vi "RVC Drive to Pose Maneuver.vi"() -> ()   [LabVIEW 2017]
uses:
  <vilib>/Simulation/Scripting/Companion Diagram/SimConfigNode/SimParams.ctl
  <vilib>/Simulation/Scripting/Companion Diagram/SimConfigNode/_simSolvers.ctl
  <vilib>/Simulation/Implementation/Shared/SIMSCR Execution Mode.ctl
  <vilib>/Simulation/Param Hierarchy/Typedefs/SIMPH Param Control Actions.ctl
  <vilib>/Simulation/Scripting/Editor Utilities/SIM subVI tag data.ctl
  <vilib>/Simulation/Scripting/Editor Utilities/SIM subVI execution type.ctl
  <vilib>/Simulation/Implementation/Shared/NILVSim_ParamChanged.vi
  <vilib>/Simulation/Implementation/Shared/NILVSIM_BeginStep.vi
  <vilib>/Simulation/Utility/Implementation/SIM Time.vi
  <vilib>/Simulation/Utility/Implementation/NILVSim Collector.llb/SIM Collector (vector).vi
  <vilib>/Simulation/SignalArithmetic/Implementation/NILVSim Gain.llb/SIM Gain (scalar).vi
  <vilib>/Simulation/Utility/Implementation/SIM Halt.vi
  <vilib>/Simulation/Utility/Implementation/NILVSim Collector.llb/SIM Collector (scalar).vi
  <vilib>/Simulation/Implementation/Shared/SIM Fire Discrete SubVI.vi
  <vilib>/Simulation/Implementation/Shared/NILVSim_Manager.vi
  <vilib>/Utility/error.llb/Clear Errors.vi
  <vilib>/Simulation/Implementation/Shared/NILVSim_FinalizeModel.vi
  <vilib>/Simulation/Utility/Implementation/NILVSim Collector.llb/NILVSim Collector core (vector).vi
  <vilib>/Simulation/Utility/Implementation/NILVSim Collector.llb/NILVSim Collector core (scalar).vi
  <vilib>/Simulation/Implementation/Shared/SIM Fire Discrete SubVI (Core).vi
  <vilib>/Simulation/Implementation/Shared/SIM Unbundle Sim Info.vi
  <vilib>/Simulation/Implementation/Shared/NILVSim_Initialize.vi
  <vilib>/Simulation/Utility/Implementation/NILVSim Get Time and IsAcceptedStep.vi
  subVIs/2D Animation.vi
  subVIs/RVC To Polar.vi
  subVIs/2D Animate Rotating Wheel.vi
  <vilib>/Simulation/Implementation/Shared/SIMSH Read Queue.vi
  <vilib>/Simulation/Implementation/Shared/NILVSim_GetModelError.vi
  <vilib>/Simulation/Implementation/Shared/SIM Bundle Sim Info.vi
  <vilib>/Simulation/Scripting/Companion Diagram/SimConfigNode/SimDog.xnode
  SIM Bicycle.vi
  <vilib>/Simulation/Implementation/XNodeFramework/SimXNode/SimX.xnode
  <vilib>/Simulation/Implementation/Shared/NI_SIM_Implementation.lvlib
panel:
  out "Velocity":cluster{"Time":dbl[], "Signal":dbl[]}[](graph)
  out "Steering":cluster{"Time":dbl[], "Signal":dbl[]}[](graph)
  out "velocity":dbl(knob)=1.0 scale=0.0..10.0
  out "Drive to Pose":cluster{"Time":dbl[], "Signal":dbl[]}[](graph)
  out "Position":cluster{"x":dbl, "y":dbl, "theta":dbl}
  out "Steering Angle":dbl format="%.2f"
  out "Steering Angle":picture
  in  "Pose":dbl[](array[numeric])=[5.0, 5.0, 1.57]
  out "Map Floor":picture
  # "Velocity"
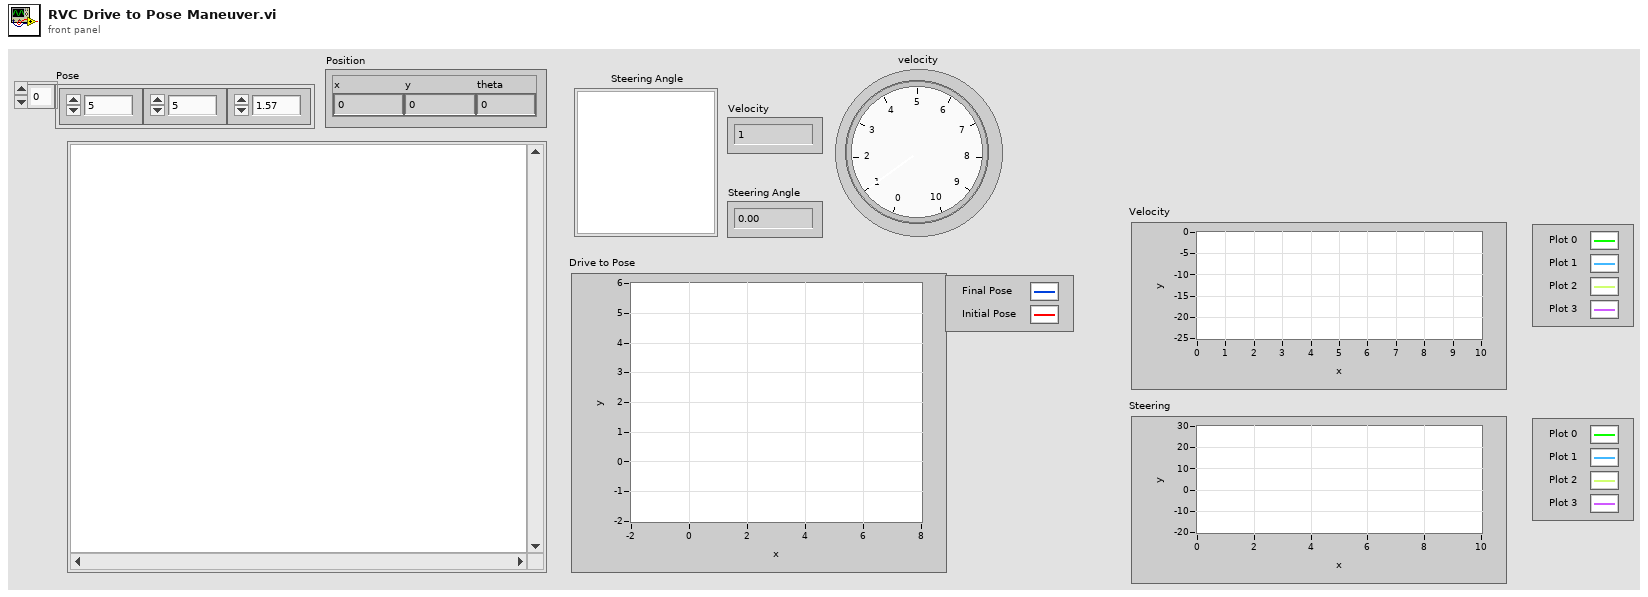
[diagram p1: front panel]
types:
  T1 = typedef "SIMSCR Execution Mode.ctl" = enum16{"Simulate to Completion", "Single Time-Step Simulation (Fixed Step Only)"}
  T2 = typedef "SIMPH Param Control Actions.ctl" = enum16{"get params", "set params"}
  T3 = typedef "SIM subVI tag data.ctl" = cluster{"period":dbl, "skew":dbl, "Simulation execution type":T4}
  T4 = typedef "SIM subVI execution type.ctl" = enum16{"Function call", "Discrete", "Continuous", "Initialization only", "Final step only"}
  T5 = cluster{"SIMSH Sim Time":dbl, "Build Array 2":cluster{"appended array":dbl[]}, "Divide 2":cluster{"x/y":dbl}, "Sine & Cosine":cluster{"sin(x)":dbl, "cos(x)":dbl}, "initial condition":dbl[], "Index Array 4":cluster{"element":dbl}, "vel limit":cluster{"output":dbl}, "steering angle limit":cluster{"output":dbl}, "acceleration limit":cluster{"output":dbl}, "Product":cluster{"Result":dbl[]}, "Build Array":cluster{"appended array":dbl[]}, "Integrator":cluster{"output":dbl[]}}
  T6 = typedef "SimParams.ctl" = cluster{"Initial Time (s)":dbl, "Final Time (s)":dbl, "Step Size (s)":dbl, "ODE Solver":T7, "Minimum Step Size (s)":dbl, "Maximum Step Size (s)":dbl, "Relative Tolerance":dbl, "Absolute Tolerance":dbl, "Software Timing":bool, "Initial Step Size (s)":dbl, "Automatic Fixed Step Size?":bool, "Automatic Discrete Step Size?":bool, "Discrete Step Size (s)":dbl, "Calculate using Time Step":bool, "Solver Wired?":bool, "Prev.Frm.Expected End":u64, "Prev.Frm.Actual End":u64, "Prev.Frm.Finished Late?":bool, "Prev.Iter.Expected End":u64, "Prev.Iter.Actual End":u64, "Prev.Iter.Finished Late?":bool, "Expected Iteration Start":u64, "Actual Iteration Start":u64, "Expected Frame Start":u64, "Actual Frame Start":u64, "Source Name":string, "Name":string, "Period":i64, "Deadline":i64, "Offset":i64, "Start":i64, "Priority":i32, "Timeout":i32, "Processor":i32, "Mode":enum32{"No Change", "Process missed periods, maintain original phase", "Discard missed periods, maintain original phase", "Process missed periods, ignore original phase", "Discard missed periods, ignore original phase"}, "Wakeup reason":enum32{"Normal", "Aborted", "Asynchronous wakeup", "Timing source error", "Timed loop error", "Timeout"}, "Error":errorcluster, "Source Type":string, "Secondary Source Type":string, "Global End Time":u64, "Global Start Time":u64, "Full Solver Reset":bool, "Execution Mode":T1, "Nan/Inf Check":bool, "Custom Solver Library":string, "Solver Is Variable":bool, "custom solver name":string, "Signal Collection Decimation":u32}
  T7 = typedef "_simSolvers.ctl" = enum16{"Runge-Kutta 1 (Euler)", "Runge-Kutta 2", "Runge-Kutta 3", "Runge-Kutta 4", "Runge-Kutta 23 (variable)", "Runge-Kutta 45 (variable)", "BDF (variable)", "Adams-Moulton (variable)", "Rosenbrock (variable)", "Discrete States Only", "SDIRK 4 (variable)", "Radau 5 (variable)", "Radau 9 (variable)", "Radau 13 (variable)", "Radau [Variable Order] (variable)", "Gear's Method (variable)", "Linearizer", "State Query", "Trim Eval", "Custom Solver"}
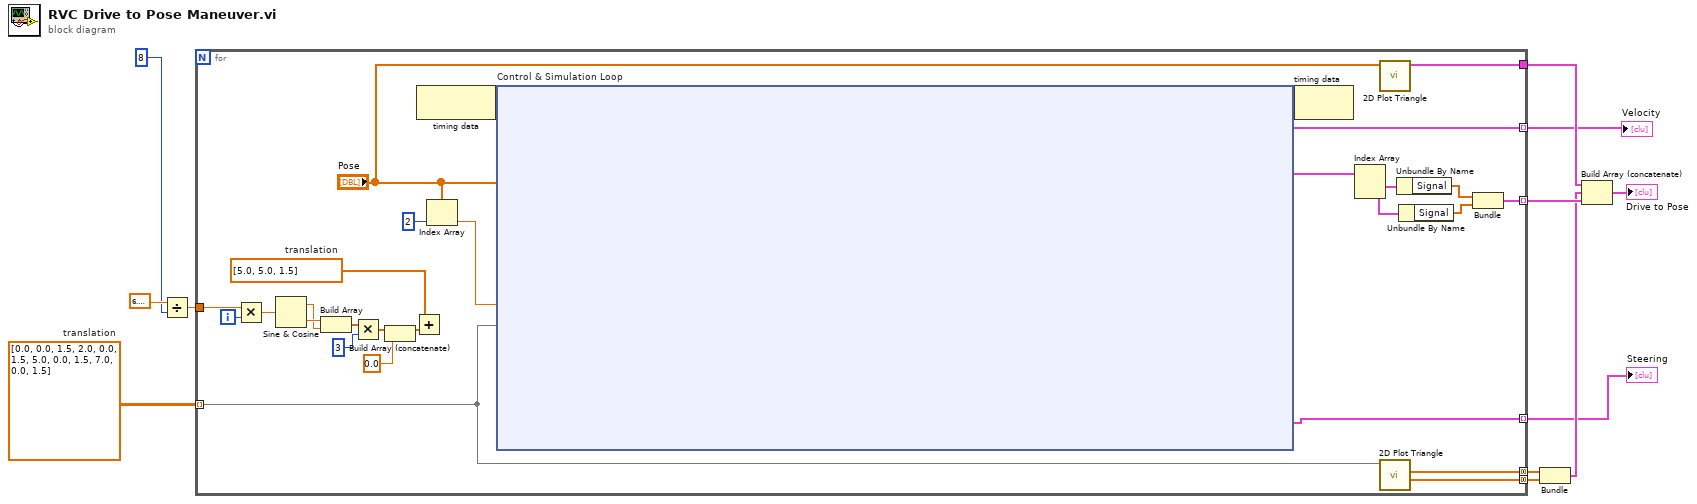
[diagram p0: block diagram]
diagram:
  w1 = dbl[][] [[0.0, 0.0, 1.5], [2.0, 0.0, 1.5], [5.0, 0.0, 1.5], [7.0, 0.0, 1.5]]  # translation
  n1 = Divide(x=6.283185307179586, y=8) -> (x/y=w9:dbl)
  n2 = for {
    tunnel: [w31] -> w12 mode=indexing
    tunnel: w9 -> [w27]
    tunnel: [w23] -> w7 mode=concatenating
    tunnel: [w22] -> w6 mode=concatenating
    tunnel: [w19] -> w4
    tunnel: [w15] -> w3 mode=indexing
    tunnel: [w14] -> w2 mode=indexing
    tunnel: w1 -> [w13] mode=indexing
    i -> [w28]
    w21 = dbl[] [5.0, 5.0, 1.5]  # translation
    n3 = Multiply(x=w27, y=w28) -> (x*y=w24:dbl)
    n4 = Sine & Cosine(0:w24) -> (1:w29:dbl, 2:w30:dbl)
    n5 = Build Array(w30, w29) -> (w38:dbl[])
    n6 = Multiply(x=w38, y=3) -> (x*y=w37:dbl[])
    n7 = Build Array (concatenate)(w37, 0.0) -> (w25:dbl[])
    n8 = Add(x=w21, y=w25) -> ()  [unwired: 1 out]
    n9 = node-c288() -> (w40:variant)  [unwired: 1 in]
    n10 = Index Array(array="Pose", index=2) -> (element=w16:dbl)
    n11 = node-c254 "Control & Simulation Loop"(w40, w13, "Pose", w16) -> (w39:variant, w36:cluster{"Time":dbl[], "Signal":dbl[]}[], w15:cluster{"Time":dbl[], "Signal":dbl[]}, w14:cluster{"Time":dbl[], "Signal":dbl[]})
    n12 = node-c288(w39) -> ()  [unwired: 1 out]
    n13 = Index Array(array=w36) -> (element #1=w35:cluster{"Time":dbl[], "Signal":dbl[]}, element #2=w34:cluster{"Time":dbl[], "Signal":dbl[]})  [unwired: 2 in]
    n14 = call "2D Plot Triangle.vi"("appended array"="Pose") -> ("output cluster"=w19:cluster{dbl[], dbl[]})  [unwired: 8 in, 2 out]
    n15 = call "2D Plot Triangle.vi"("appended array"=w13) -> ("Y"=w22:dbl[], "X"=w23:dbl[])  [unwired: 8 in, 1 out]
    n16 = Unbundle By Name(w35) -> ("Signal"=w33:dbl[])
    n17 = Unbundle By Name(w34) -> ("Signal"=w32:dbl[])
    n18 = Bundle("Signal"=w33, "Signal"=w32) -> (w31:cluster{"Signal":dbl[], "Signal":dbl[]})  [unwired: 1 in]
  }
  "Steering" <- w3
  "Velocity" <- w2
  n19 = Bundle("X"=w7, "Y"=w6) -> (w5:cluster{"X":dbl[], "Y":dbl[]})  [unwired: 1 in]
  n20 = Build Array (concatenate)(w4, w5, w12) -> (→"Drive to Pose":cluster{"Signal":dbl[], "Signal":dbl[]}[])
